vi "status.vi"(7 "resetFlag":i32, 8 "error in (no error)":errorcluster, 9 "pHighwater":i32, 10 "pCurrent":i32, 11 "op":i32) -> (0 "error out":errorcluster, 1 "pHighwater out":i32, 2 "pCurrent out":i32, 3 "function return":i32)   [LabVIEW 2020, in "sqlite3.lvlib"]
uses:
  sqlite3.lvlib
  errstr.vi
  bin/sqlite3_64.dll
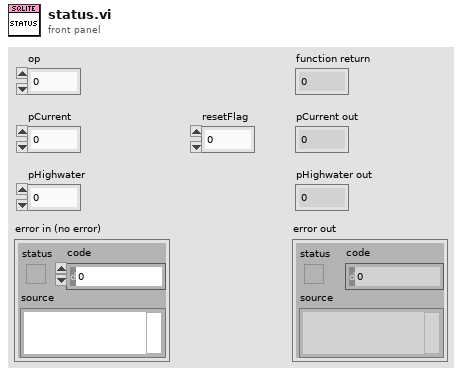
[diagram p1: front panel]
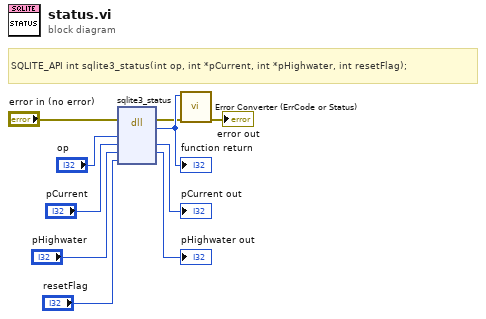
[diagram p0: block diagram]
diagram:
  # "SQLITE_API int sqlite3_status(int op, int *pCurrent, int *pHighwater, int resetFlag);"
  n1 = dll-call lib="C:/Users/Fred.Guo/Desktop/Database-configuration/externals/sqlite3/Source/bin/sqlite3_*.*" fn="sqlite3_status"(error in="error in (no error)", "op"="op", "pCurrent"="pCurrent", "pHighwater"="pHighwater", "resetFlag"="resetFlag") -> (error out=w2:errorcluster, w10:i32, "pCurrent"=→"pCurrent out":i32, "pHighwater"=→"pHighwater out":i32)  [unwired: 4 in, 1 out]
  "function return" <- w10
  n2 = call "Error Converter (ErrCode or Status).vi"("error in (no error)"=w2, "error code"=w10) -> ("error out"=→"error out":errorcluster)  [unwired: 9 in]
